vi "Write Strings to File.vi"(8 "Error In":errorcluster, 9 "Section Name":string, 10 "Array of Strings":string[](array[string]), 11 "Path":path) -> (0 "Error Out":errorcluster)   [LabVIEW 2020]
doc: "This VI was created for use with the Read/Write Cluster VIs. It writes the cluster element strings to the specified section in an INI file without editing any other sections.\n\nFreeware from Moore Good Ideas, www.mooregoodideas.com. Do not remove this line."
uses:
  Suppress Error Code - Scalar.vi
panel:
  out "unsigned byte array":u8[](array[numeric])
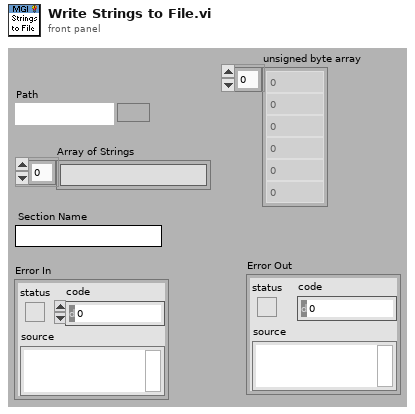
[diagram p1: front panel]
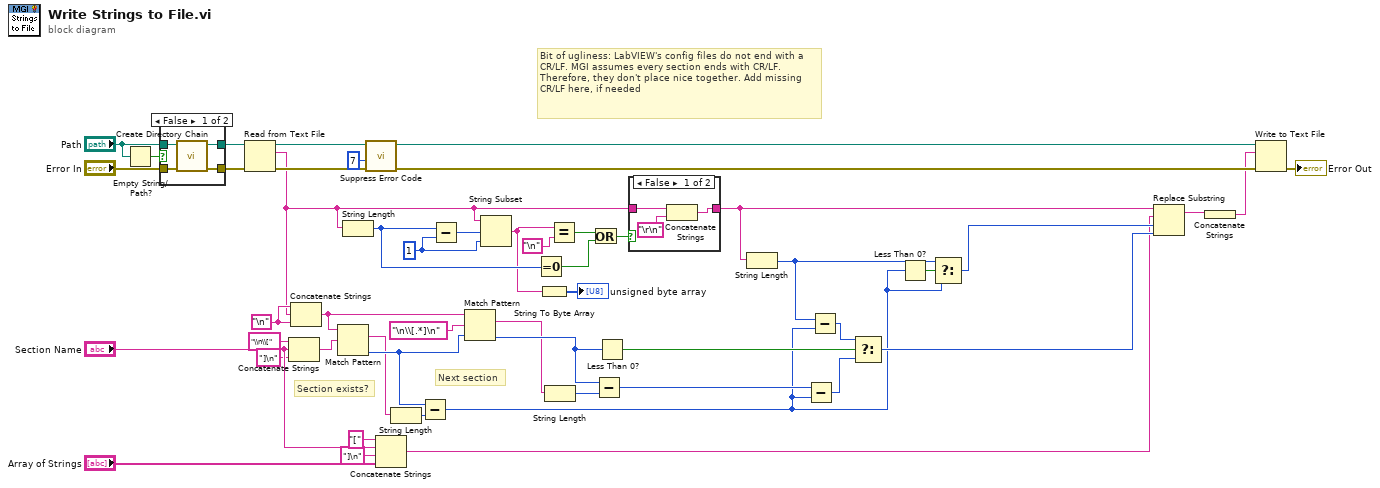
[diagram p0: block diagram]
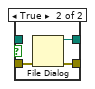
[diagram p3: hidden frame]
diagram:
  w3 = 1
  w18 = "\n"
  # "Bit of ugliness: LabVIEW's config files do not end with a CR/LF. MGI assumes every section ends with CR/LF. Therefore, they don't place nice together. Add missing CR/LF here, if needed"
  # "Next section"
  # "Section exists?"
  n1 = Empty String/Path?(string/path="Path") -> (empty?=w19:bool)
  n2 = case shown="False" w19 {
    tunnel: "Error In" -> [w52 w55]
    tunnel: [w51 w54] -> w24
    tunnel: [w50 w53] -> w23
    tunnel: "Path" -> [w49 _]
    frame False {
      n3 = call "Create Directory Chain.vi"("Error In"=w52, "Path"=w49) -> ("Error Out"=w51:errorcluster, "Duplicate Path"=w50:path)  [unwired: 8 in]
    }
    frame True {
      n4 = File Dialog(8:w55) -> (0:w54:errorcluster, 3:w53:path)  [unwired: 6 in, 2 out]
    }
  }
  n5 = Read from Text File(file (use dialog)=w23, error in=w24) -> (text=w9:string, error out=w30:errorcluster)  [unwired: 2 in, 2 out]
  n6 = Concatenate Strings("\\n\\[" ("string"), "Section Name", "]\n" ("string")) -> (w43:string)
  n7 = Concatenate Strings(w18, w9, w18) -> (w21:string)
  n8 = Match Pattern(string=w21, regular expression=w43) -> (match substring=w33:string, offset past match=w37:i32)  [unwired: 1 in, 2 out]
  n9 = String Length(string=w9) -> (length=w6:i32)
  n10 = call-poly "Suppress Error Code.vi"("Error In"=w30, "Error Code"=7) -> ("Error Out"=w47:errorcluster)  [unwired: 8 in, 1 out]
  n11 = Concatenate Strings("[" ("string"), "Section Name", "]\n" ("string"), "Array of Strings") -> (w14:string)
  n12 = String Length(string=w33) -> (length=w32:i32)
  n13 = Subtract(x=w37, y=w32) -> (x-y=w13:i32)
  n14 = Subtract(x=w6, y=w3) -> (x-y=w12:i32)
  n15 = Match Pattern(string=w21, regular expression="\n\\[.*]\n", offset (0)=w37) -> (match substring=w35:string, offset past match=w40:i32)  [unwired: 2 out]
  n16 = String Subset(string=w9, offset (0)=w12, length (rest)=w3) -> (substring=w2:string)
  n17 = Equal To 0?(x=w6) -> (x = 0?=w4:bool)
  n18 = String To Byte Array(string=w2) -> (unsigned byte array=→"unsigned byte array":u8[])
  n19 = String Length(string=w35) -> (length=w34:i32)
  n20 = Equal?(x=w2, y="\n") -> (x = y?=w10:bool)
  n21 = Or(x=w10, y=w4) -> (x .or. y?=w5:bool)
  n22 = Subtract(x=w40, y=w34) -> (x-y=w36:i32)
  n23 = Less Than 0?(x=w40) -> (x < 0?=w39:bool)
  n24 = case shown="False" w5 {
    tunnel: w9 -> [w57 w59]
    tunnel: [w56 w59] -> w8
    frame False {
      n25 = Concatenate Strings(w57, "\r\n") -> (w56:string)
    }
    frame True {
    }
  }
  n26 = String Length(string=w8) -> (length=w7:i32)
  n27 = Subtract(x=w36, y=w13) -> (x-y=w41:i32)
  n28 = Subtract(x=w7, y=w13) -> (x-y=w42:i32)
  n29 = Select(t=w42, s=w39, f=w41) -> (s? t:f=w38:i32)
  n30 = Less Than 0?(x=w13) -> (x < 0?=w22:bool)
  n31 = Select(t=w7, s=w22, f=w13) -> (s? t:f=w15:i32)
  n32 = Replace Substring(2:w38, 3:w15, 4:w14, 5:w8) -> (1:w17:string)  [unwired: 1 out]
  n33 = Concatenate Strings(w17) -> (w16:string)
  n34 = Write to Text File(file (use dialog)=w23, text=w16, error in=w47) -> (error out=→"Error Out":errorcluster)  [unwired: 1 in, 2 out]
